vi "Add TypeDefs to System Explorer.vi"(6 "SE Path Cluster In":T3, 7 "Pages Properties":T1[](array[typedef]), 8 "error in":errorcluster) -> (0 "error out":errorcluster, 4 "SE Path Cluster In":T3)   [LabVIEW 2026, in "NIVS_CDEW_MetaDataObj.lvclass"]
uses:
  NIVS_CDEW_MetaDataObj.lvclass
  Types/Page Properties.ctl
  Types/Page Types.ctl
  7e2e5944-2803-4f61-b14d-e9b6cd5ae37f.vi
  NIVS_CDEW_MetaDataObj.lvclass/NIVS_CDEW_MetaDataObj.ctl
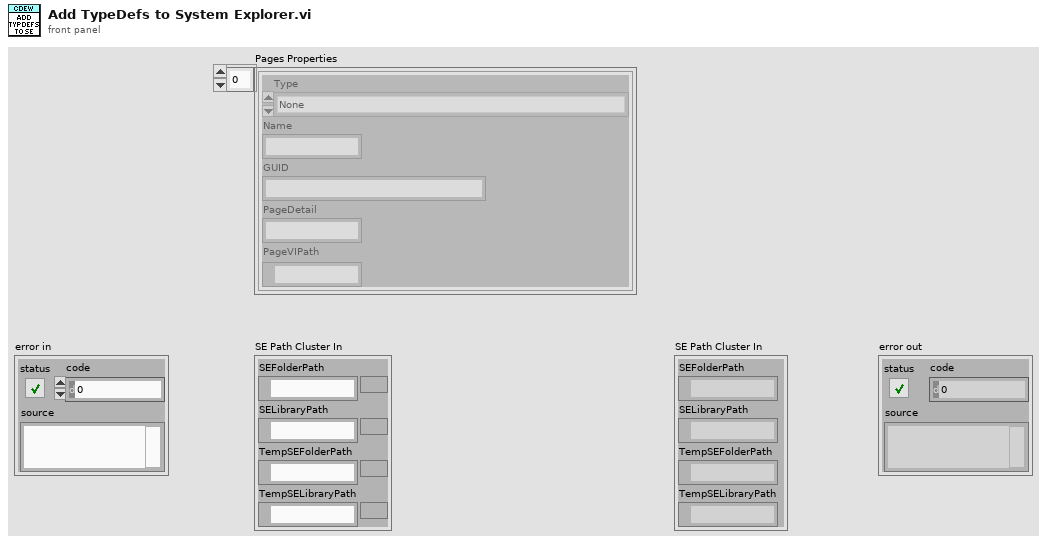
[diagram p1: front panel]
types:
  T1 = typedef "NIVS_CDEW_MetaDataObj.lvclass/Page Properties.ctl" = cluster{"Type":T2, "Name":string, "GUID":string, "PageDetail":string, "PageVIPath":path}
  T2 = typedef "NIVS_CDEW_MetaDataObj.lvclass/Page Types.ctl" = enum16{"None", "CustomDevice", "Channel", "Waveform", "Section", "DynamicChannel", "DynamicWaveform", "DynamicSection"}
  T3 = cluster{"SEFolderPath":path, "SELibraryPath":path, "TempSEFolderPath":path, "TempSELibraryPath":path}
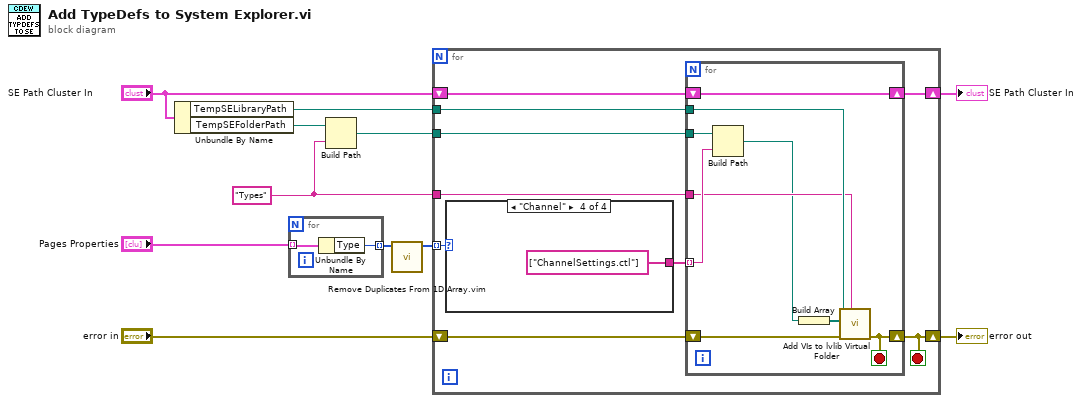
[diagram p0: block diagram]
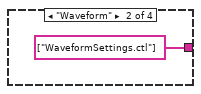
[diagram p3: hidden frame]
diagram:
  w3 = "Types" ("Virtual Folder Name")
  n1 = Unbundle By Name("SE Path Cluster In") -> ("TempSELibraryPath"=w1:path, "TempSEFolderPath"=w2:path)
  n2 = for {
    tunnel: "Pages Properties" -> [w13] mode=indexing
    tunnel: [w12] -> w7 mode=indexing
    n3 = Unbundle By Name(w13) -> ("Type"=w12:T2)
  }
  n4 = Build Path(base path=w2, name or relative path=w3) -> (appended path=w4:path)
  n5 = call "Remove Duplicates From 1D Array.vim"("array"=w7) -> ("array with duplicates removed"=w6:T2[])  [unwired: 10 in]
  n6 = for {
    shift-right: [w17] -> w10
    shift-left: "error in" -> [w22]
    shift-right: [w20] -> w11
    shift-left: "SE Path Cluster In" -> [w21]
    tunnel: w6 -> [w18] mode=indexing
    tunnel: w1 -> [w16]
    tunnel: w4 -> [w15]
    tunnel: w3 -> [w14]
    stop <- w17 stop-if-true
    n7 = case shown="\"Channel\"" w18 {
      tunnel: [_ string[] ["WaveformSettings.ctl"] _ string[] ["ChannelSettings.ctl"]] -> w19
      frame "None", "CustomDevice", "DynamicChannel".."DynamicSection" {
      }
      frame "Waveform" {
      }
      frame "Section" {
      }
      frame "Channel" {
      }
    }
    n8 = for {
      shift-right: [w28] -> w17
      shift-left: w22 -> [w29]
      shift-right: [w31] -> w20
      shift-left: w21 -> [w31]
      tunnel: w19 -> [w25] mode=indexing
      tunnel: w16 -> [w27]
      tunnel: w15 -> [w26]
      tunnel: w14 -> [w24]
      stop <- w28 stop-if-true
      n9 = Build Path(base path=w26, name or relative path=w25) -> (appended path=w23:path)
      n10 = Build Array(w23) -> (w30:path[])
      n11 = call "Add VIs to lvlib Virtual Folder.vi"("Virtual Folder Name"=w24, "error in"=w29, "VIs to add"=w30, "lvlib Path"=w27) -> ("error out"=w28:errorcluster)  [unwired: 7 in]
    }
  }
  "SE Path Cluster In" <- w11
  "error out" <- w10
